vi "GenerateApriltag25h9.vi"(8 "error in (no error)":errorcluster, 11 "ID":i32) -> (0 "error out":errorcluster, 3 "Tag Pixel Array":u8[][](array[numeric]) format="%.0x")   [LabVIEW 2020, in "g_ar_toolkit.feature_detection.lvlib"]
uses:
  g_ar_toolkit.feature_detection.lvlib
  TagIDOutOfRangeError.vi
  <vilib>/Utility/error.llb/Error Cluster From Error Code.vi
  TagLayoutConvert.vi
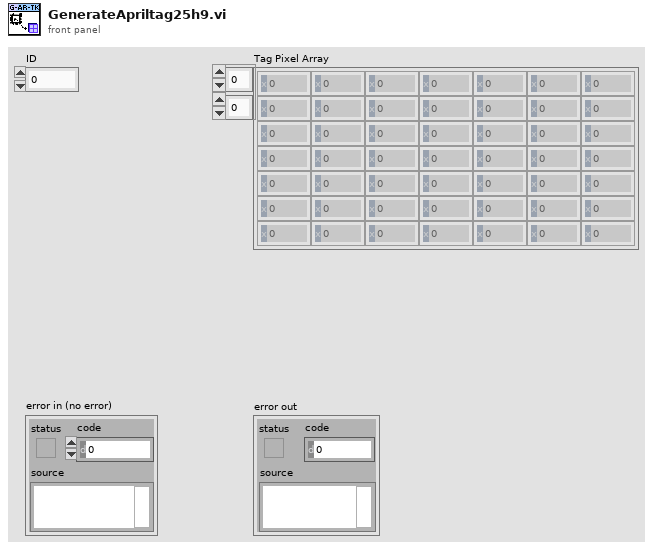
[diagram p1: front panel]
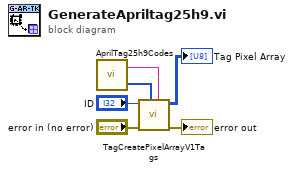
[diagram p0: block diagram]
diagram:
  n1 = call "AprilTag25h9Codes.vi"() -> ("Codes"=w3:i64[], "Layout"=w1:string)  [unwired: 2 in]
  n2 = call "TagCreatePixelArrayV1Tags.vi"("Layout"=w1, "Codes"=w3, "error in (no error)"="error in (no error)", "ID"="ID") -> ("error out"=→"error out":errorcluster, "Pixels"=→"Tag Pixel Array":u8[][])  [unwired: 6 in]
